vi "FPGA Circular Buffer.vi"(8 "request data":bool, 10 "send data":bool, 11 "stream.state 0":T1) -> (1 "Read Pointer":u32, 2 "send data out":bool, 3 "Write Pointer":u32)   [LabVIEW 2014]
uses:
  <instrlib>/_niInstr/Streaming/v1/Common/Stream State.ctl
  <instrlib>/_niInstr/Streaming/v1/Common/niInstr Streaming v1 Common.lvlib
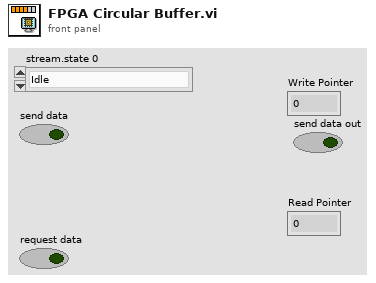
[diagram p1: front panel]
types:
  T1 = typedef "niInstr Streaming v1 Common.lvlib/Stream State.ctl" = enum8{"Idle", "Finite Transfer", "Continuous", "Done", "Error", "Not Ready", "Cancel"}
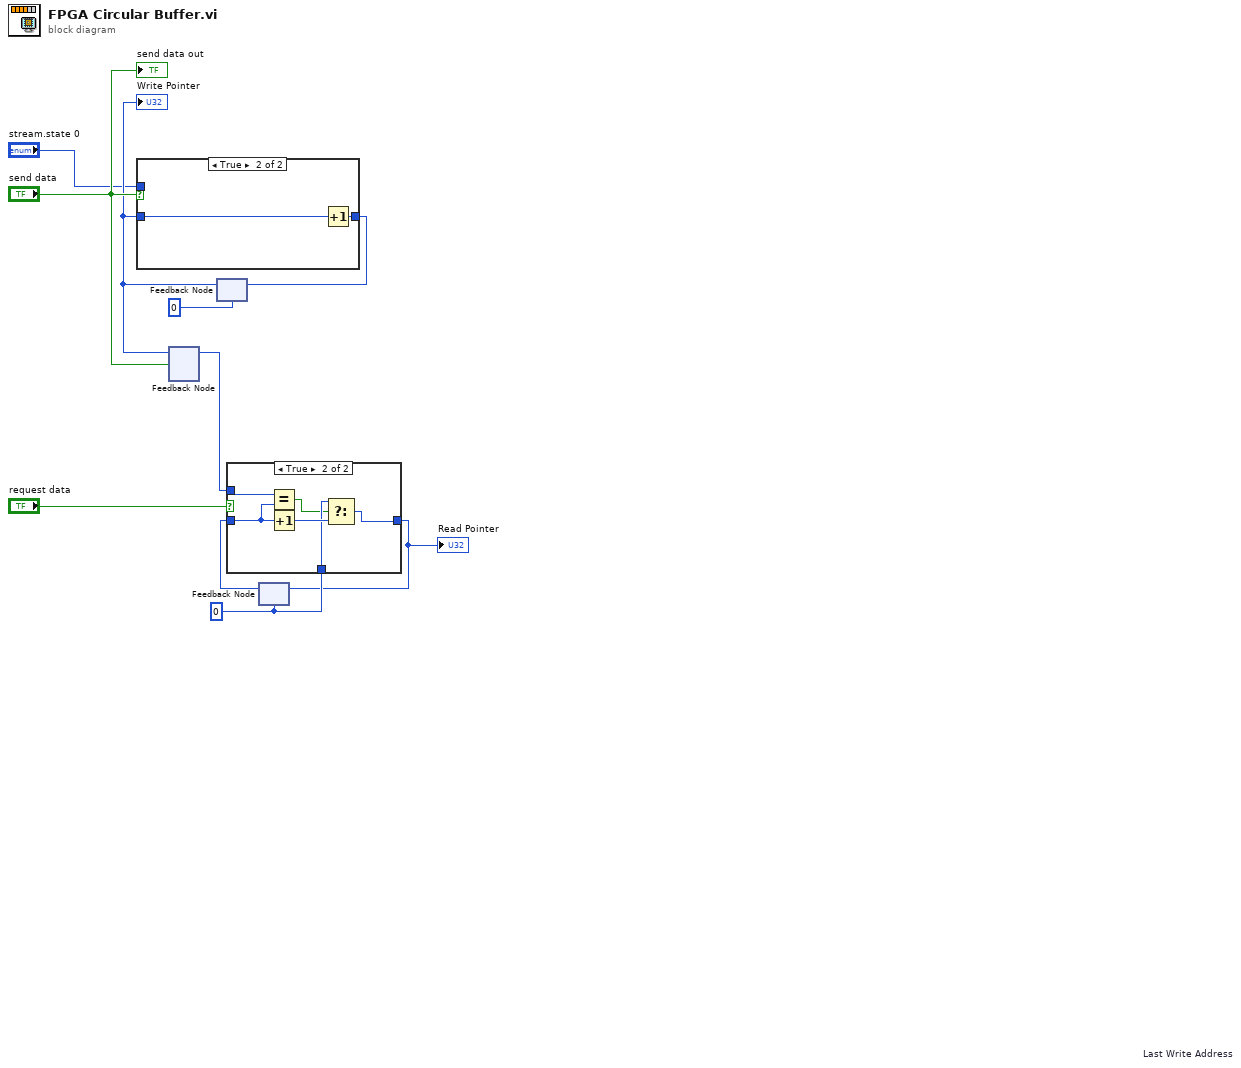
[diagram p0: block diagram]
diagram:
  w8 = u32 0
  n1 = feedback #1 "Last Write Address"() -> (w9:u32)  [unwired: 1 in]
  n2 = feedback #2(u32 0) -> (w6:u32)
  "Write Pointer" <- w6
  n3 = case shown="True" "send data" {
    tunnel: w6 -> [w12 w16]
    tunnel: [w11 w15] -> w2
    tunnel: "stream.state 0" -> [w13 _]
    frame False {
      n4 = case shown="\"Finite Transfer\", Default" w13 {
        tunnel: w12 -> [_ w14]
        tunnel: [_ w14] -> w11
        frame "Idle" {
        }
        frame "Finite Transfer", Default {
        }
      }
    }
    frame True {
      n5 = Increment(x=w16) -> (x+1=w15:u32)
    }
  }
  n6 = feedback-in #1(w6, "send data") -> ()
  n7 = feedback-in #2(w2) -> ()
  n8 = feedback #3(w8) -> (w4:u32)
  n9 = case shown="True" "request data" {
    tunnel: w4 -> [_ w19]
    tunnel: [_ w21] -> w5
    tunnel: w8 -> [_ w20]
    tunnel: w9 -> [_ w18]
    frame False {
    }
    frame True {
      n10 = Equal?(x=w18, y=w19) -> (x = y?=w17:bool)
      n11 = Increment(x=w19) -> (x+1=w22:u32)
      n12 = Select(t=w20, s=w17, f=w22) -> (s? t:f=w21:u32)
    }
  }
  "Read Pointer" <- w5
  n13 = feedback-in #3(w5) -> ()
  "send data out" <- "send data"
